vi "Get Adjusted Ring Exposure Times.vi"(8 "error in (no error)":errorcluster, 10 "fptimes":sgl, 11 "inumTimes":i32) -> (0 "error out":errorcluster, 2 "fptimes out":sgl, 3 "function return":u32)   [LabVIEW 2014, in "atmcd32d.lvlib"]
doc: "unsigned int WINAPI GetAdjustedRingExposureTimes(int inumTimes, float * fptimes);"
uses:
  atmcd32d.lvlib
  atmcd32d.dll
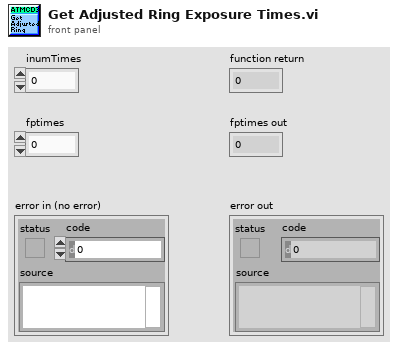
[diagram p1: front panel]
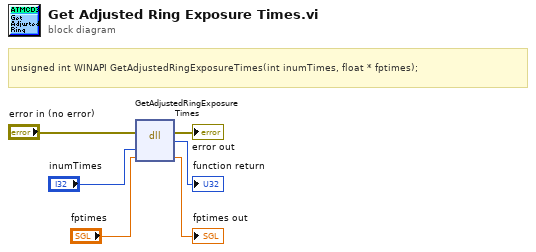
[diagram p0: block diagram]
diagram:
  # "unsigned int WINAPI GetAdjustedRingExposureTimes(int inumTimes, float * fptimes);"
  n1 = dll-call lib="C:/Users/Bakir/Documents/Lambda2-Testing/lib/Andorlib/atmcd32d.*" fn="GetAdjustedRingExposureTimes"(error in="error in (no error)", "inumTimes"="inumTimes", "fptimes"="fptimes") -> (error out=→"error out":errorcluster, →"function return":u32, "fptimes"=→"fptimes out":sgl)  [unwired: 3 in, 1 out]
